vi "RTP_RTSP - DESCRIBE - METHOD.vi"(0 "address":string, 1 "port":u16=554, 5 "uid":string, 7 "pwd":string, 9 "timeout ms (1000)":i32=1000, 11 "error in (no error)":errorcluster, 12 "Stream File":string) -> (4 "RTSP Session":T1, 15 "error out":errorcluster)   [LabVIEW 2014]
uses:
  RTSP Session.ctl
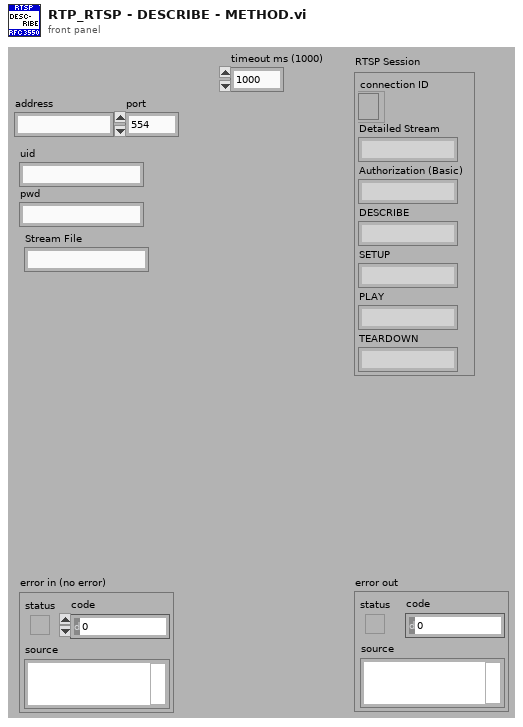
[diagram p1: front panel]
types:
  T1 = typedef "RTSP Session.ctl" = cluster{"connection ID":refnum<k5>, "Authorization (Basic)":string, "Detailed Stream":string, "DESCRIBE":string, "SETUP":string, "PLAY":string, "TEARDOWN":string}
  T2 = enum16{"Standard", "Buffered", "CRLF", "Immediate"}
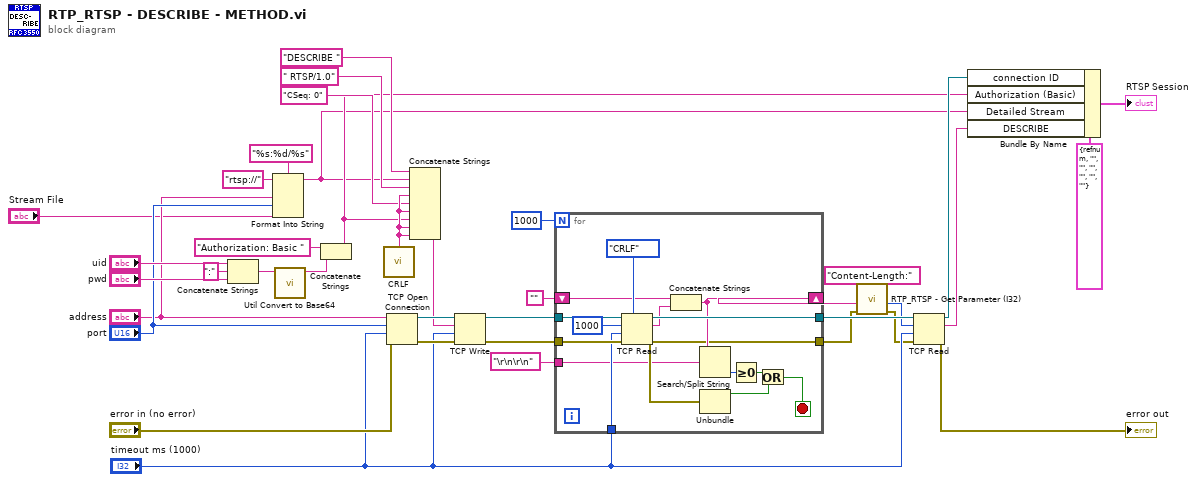
[diagram p0: block diagram]
diagram:
  n1 = Concatenate Strings("uid", ":" ("string"), "pwd") -> (w16:string)
  n2 = Format Into String(format string="%s:%d/%s", initial string="rtsp://", "address", "port", "Stream File") -> (resulting string=w6:string)  [unwired: 1 in, 1 out]
  n3 = call "Util Convert to Base64.vi"("String"=w16) -> ("Base64 String"=w15:string)  [unwired: 10 in]
  n4 = Concatenate Strings("Authorization: Basic ", w15) -> (w7:string)
  n5 = call "CRLF.vi"() -> ("CRLF"=w30:string)
  n6 = TCP Open Connection(address="address", remote port or service name="port", timeout ms (60000)="timeout ms (1000)", error in (no error)="error in (no error)") -> (connection ID=w38:refnum<k5>, error out=w37:errorcluster)  [unwired: 1 in]
  n7 = Concatenate Strings("DESCRIBE ", w6, " RTSP/1.0", w30, "CSeq: 0", w30, w7, w30, w30) -> (w32:string)
  n8 = TCP Write(connection ID=w38, data in=w32, error in (no error)=w37, 9:"timeout ms (1000)") -> (connection ID out=w25:refnum<k5>, error out=w24:errorcluster)  [unwired: 1 out]
  n9 = for {
    N: 1000 -> [_]
    tunnel: w24 -> [w53]
    tunnel: w25 -> [w52]
    tunnel: [w51] -> w23
    tunnel: [w43] -> w3
    shift-right: [w45] -> w5
    shift-left: "" -> [w49]
    tunnel: "timeout ms (1000)" -> [w46]
    tunnel: "\r\n\r\n" ("search string/char (-)") -> [w42]
    stop <- w39 stop-if-true
    n10 = TCP Read(connection ID=w52, bytes to read=1000, error in (no error)=w53, 7:T2."CRLF" ("mode (standard)"), 9:w46) -> (connection ID out=w51:refnum<k5>, data out=w48:string, error out=w43:errorcluster)
    n11 = Concatenate Strings(w49, w48) -> (w45:string)
    n12 = Search/Split String(string=w45, search string/char (-)=w42) -> (offset of match=w44:i32)  [unwired: 1 in, 2 out]
    n13 = Unbundle(w43) -> ("status"=w40:bool)  [unwired: 2 out]
    n14 = Greater Or Equal To 0?(x=w44) -> (x >= 0?=w41:bool)
    n15 = Or(x=w41, y=w40) -> (x .or. y?=w39:bool)
  }
  n16 = call "RTP_RTSP - Get Parameter (I32).vi"("Name"="Content-Length:", "error in"=w3, "Data"=w5) -> ("error out"=w2:errorcluster, "Parameter (I32)"=w22:i32)  [unwired: 7 in]
  n17 = TCP Read(connection ID=w23, bytes to read=w22, error in (no error)=w2, 9:"timeout ms (1000)") -> (connection ID out=w8:refnum<k5>, data out=w4:string, error out=→"error out":errorcluster)  [unwired: 1 in]
  n18 = Bundle By Name(cluster=T1 {"connection ID"=refnum, "Authorization (Basic)"="", "Detailed Stream"="", "DESCRIBE"="", "SETUP"="", "PLAY"="", "TEARDOWN"=""} ("RTSP Session"), "connection ID"=w8, "Authorization (Basic)"=w7, "Detailed Stream"=w6, "DESCRIBE"=w4) -> (→"RTSP Session":T1)
